vi "Handle Error.vi"(8 "error in (no error)":errorcluster, 11 "Base UI Component in":refnum<class "Base UI Component.lvclass">) -> (0 "error out":errorcluster, 2 "stop actor?":bool=TRUE, 3 "Base UI Component out":refnum<class "Base UI Component.lvclass">)   [LabVIEW 2017, in "Assert API Components.lvlib" / "Assert Display.lvlib" / "Base UI Component.lvlib" / "Base UI Component.lvclass"]
doc: "(<B>Filename</B>: Actor Framework.lvlib:Actor.lvclass:Handle Error.vi)\n\nDefines how the actor handles an error that occurred while processing a message. By default, this method does nothing except stop the actor."
uses:
  Base UI Component.lvclass
  Base UI Actor/Base UI Actor/Base UI Actor.lvclass
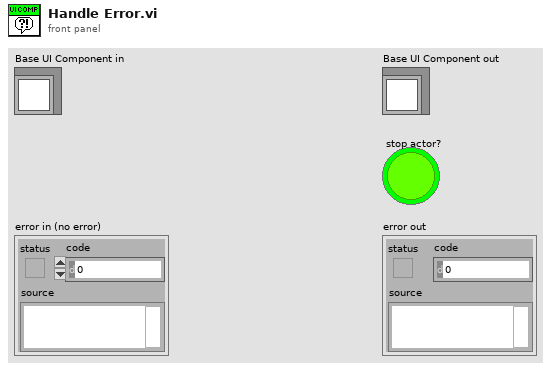
[diagram p1: front panel]
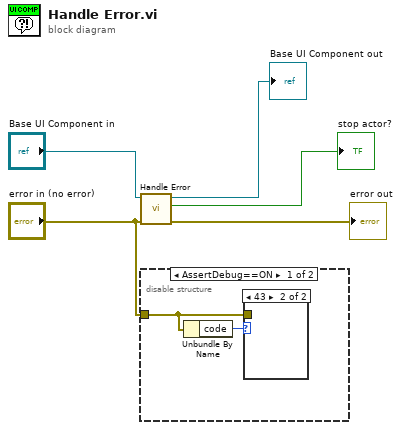
[diagram p0: block diagram]
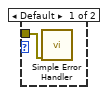
[diagram p2: hidden frame]
diagram:
  n1 = call-parent "Handle Error.vi"("error in (no error)"="error in (no error)", "Base UI Actor in"="Base UI Component in") -> ("error out"=→"error out":errorcluster, "stop actor?"=→"stop actor?":bool, "Base UI Actor out"=→"Base UI Component out":refnum<class "Base UI Component.lvclass">)  [unwired: 7 in]
  n2 = disable-structure shown="AssertDebug==ON" {
    disable-tunnel: "error in (no error)" -> [w7 _]
    frame condition #0 (active) {
      n3 = Unbundle By Name(w7) -> ("code"=w6:i32)
      n4 = case shown="43" w6 {
        tunnel: w7 -> [w8 _]
        frame Default {
          n5 = call <vilib>:"Simple Error Handler.vi"("error in (no error)"=w8) -> ()  [unwired: 4 in, 5 out]
        }
        frame 43 {
        }
      }
    }
    frame condition #1 {
    }
  }
